vi "LRMS_Scan_Test_auto.vi"() -> ()   [LabVIEW 2019]
uses:
  <instrlib>/niSwitch/niSwitch.llb/niSwitch Connect Channels (Multiple).vi
  <instrlib>/niSwitch/niSwitch.llb/niSwitch Disconnect Channels (Multiple).vi
panel:
  in  "error in":errorcluster
  out "Device List":refnum<k15>[](array[refnum])=["2526_1", "SwitchBlock1Dev1"]
  in  "Channel Index":i32
  out "Current Connection":string[](array[string])
  out "Channel Specs":string[][](array[string])
  in  "Channel List":string[](array[string])=["ch0", "ch1", "ch2", "ch3", "ch4", "ch5", "ch6"]
  in  "Connection List":path=path "C:/Users/bbrice_VM/Documents/LV Apps/LRMS/PPack_B Build/Config/Chad_Test.csv"
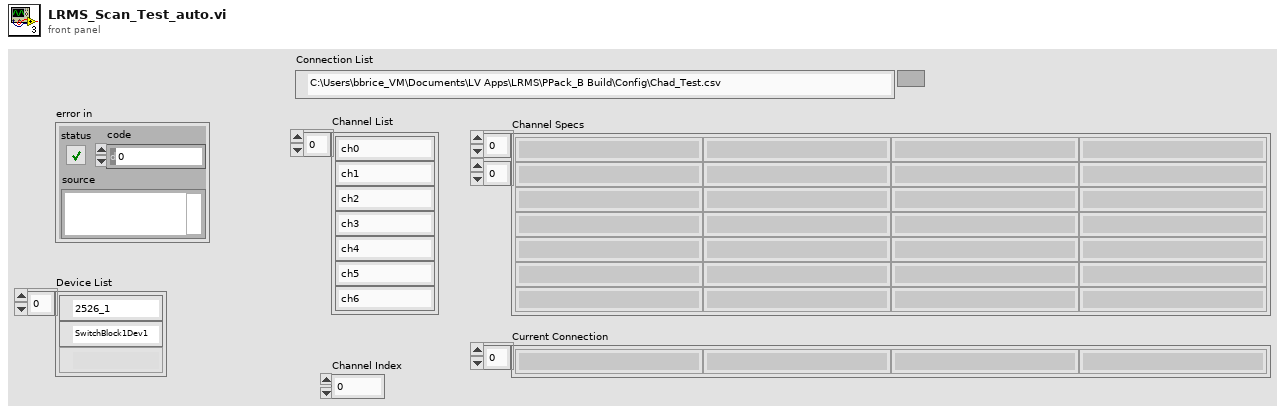
[diagram p1: front panel]
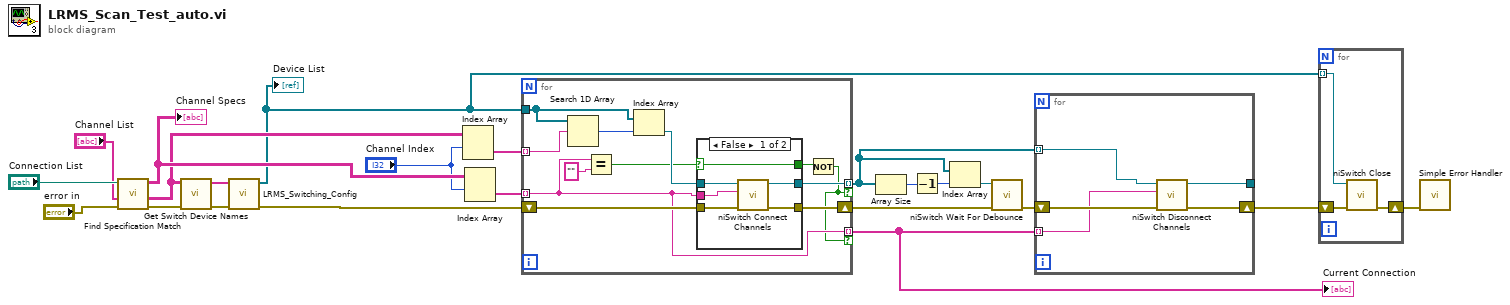
[diagram p0: block diagram]
diagram:
  n1 = call "Find Specification Match.vi"("error in (no error)"="error in", "Channel List"="Channel List", "file path (dialog if empty)"="Connection List") -> ("error out"=w16:errorcluster, "IVI Specifications"=w13:string[][], "Channel Specs"=w19:string[][])  [unwired: 5 in]
  "Channel Specs" <- w19
  n2 = call "Get Switch Device Names.vi"("IVI Specifications"=w13, "error in (no error)"=w16) -> ("Device Names"=w12:string[], "error out"=w15:errorcluster)  [unwired: 7 in]
  n3 = call "LRMS_Switching_Config.vi"("error in (no error)"=w15, "Sense MUX Devices"=w12) -> ("error out"=w11:errorcluster, "Array"=w10:refnum<k15>[])  [unwired: 8 in]
  "Device List" <- w10
  n4 = Index Array(array=w13, index (row)="Channel Index") -> (element=w8:string[])  [unwired: 1 in]
  n5 = Index Array(array=w19, index (row)="Channel Index") -> (element=w3:string[])  [unwired: 1 in]
  n6 = for {
    tunnel: w8 -> [w34] mode=indexing
    tunnel: w10 -> [w26]
    tunnel: w3 -> [w24] mode=indexing
    tunnel: [w30] -> w2 mode=indexing if=w23
    shift-right: [w29] -> w6
    shift-left: w11 -> [w31]
    tunnel: [w24] -> w17 mode=indexing if=w23
    n7 = Search 1D Array(1D array=w26, element=w34) -> (index of element=w33:i32)  [unwired: 1 in]
    n8 = Equal?(x=w24, y="") -> (x = y?=w27:bool)
    n9 = Index Array(array=w26, index=w33) -> (element=w32:refnum<k15>)
    n10 = case shown="False" w27 {
      selector: w27 -> [w35 w41]
      tunnel: w32 -> [w40 w43]
      tunnel: w31 -> [w39 w42]
      tunnel: [w38 w43] -> w30
      tunnel: [w37 w42] -> w29
      tunnel: w24 -> [w36 _]
      tunnel: [w35 w41] -> w25
      frame False {
        n11 = call-poly <instrlib>:"niSwitch Connect Channels.vi"("error in (no error)"=w39, "connection list"=w36, "instrument handle"=w40) -> ("error out"=w37:errorcluster, "instrument handle out"=w38:refnum<k15>)  [unwired: 7 in]
      }
      frame True {
      }
    }
    n12 = Not(x=w25) -> (.not. x?=w23:bool)
  }
  "Current Connection" <- w17
  n13 = Array Size(array=w2) -> (size(s)=w9:i32)
  n14 = Decrement(x=w9) -> (x-1=w4:i32)
  n15 = Index Array(array=w2, index=w4) -> (element=w1:refnum<k15>)
  n16 = call <instrlib>:"niSwitch Wait For Debounce.vi"("error in (no error)"=w6, "instrument handle"=w1) -> ("error out"=w5:errorcluster)  [unwired: 8 in, 1 out]
  n17 = for {
    tunnel: w2 -> [w48] mode=indexing
    shift-right: [w45] -> w18
    shift-left: w5 -> [w47]
    tunnel: [w46] -> _
    tunnel: w17 -> [w44] mode=indexing
    n18 = call-poly <instrlib>:"niSwitch Disconnect Channels.vi"("error in (no error)"=w47, "disconnection list"=w44, "instrument handle"=w48) -> ("error out"=w45:errorcluster, "instrument handle out"=w46:refnum<k15>)  [unwired: 7 in]
  }
  n19 = for {
    shift-right: [w50] -> w20
    shift-left: w18 -> [w51]
    tunnel: w10 -> [w49] mode=indexing
    n20 = call <instrlib>:"niSwitch Close.vi"("error in (no error)"=w51, "instrument handle"=w49) -> ("error out"=w50:errorcluster)  [unwired: 9 in]
  }
  n21 = call <vilib>:"Simple Error Handler.vi"("error in (no error)"=w20) -> ()  [unwired: 4 in, 5 out]
